vi "TEST-Get DataType Description String2.vi"() -> ()   [LabVIEW 2017]
panel:
  out "x = y?":bool[](array[boolean])
  out "unsigned byte array 2":u8[](array[numeric])
  out "unsigned byte array":u8[](array[numeric])
  out "variant 2":variant
  out "variant":variant
  out "Type 7":string
  out "Type 6":string
  out "Type 5":string
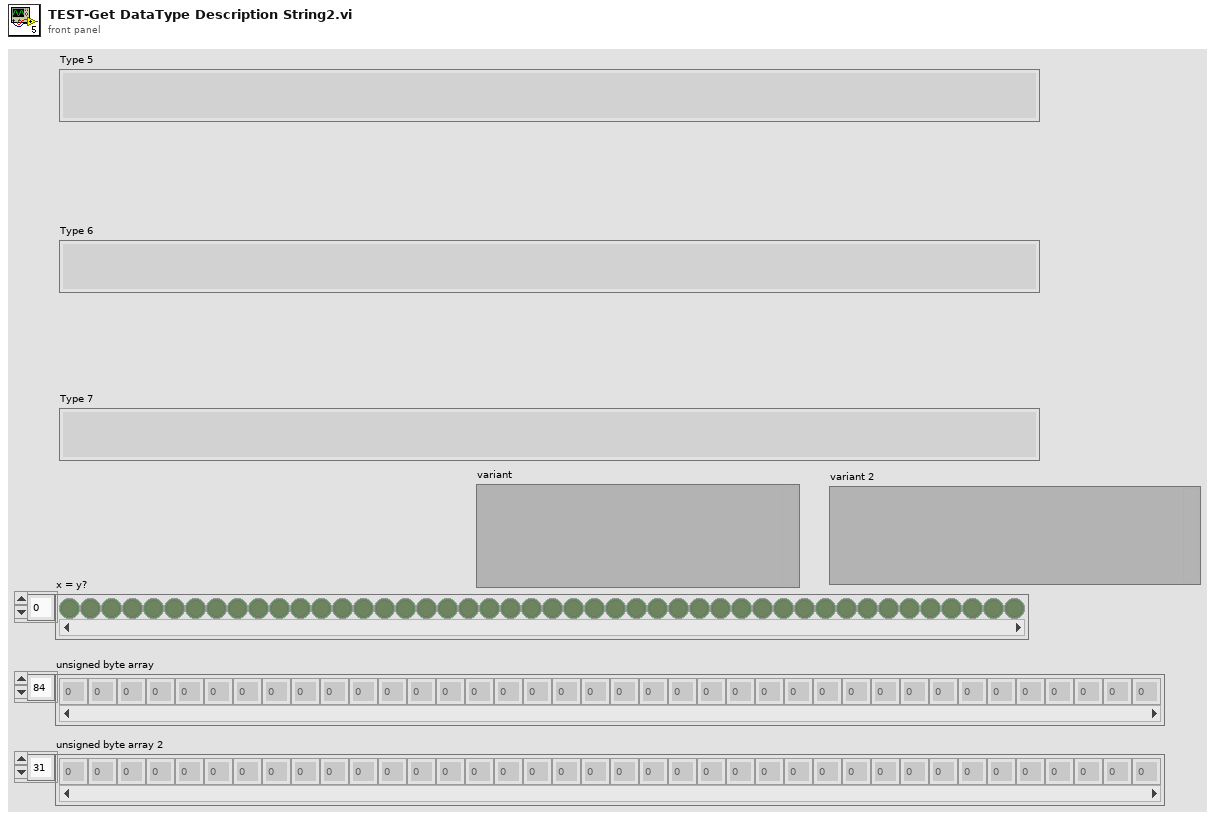
[diagram p1: front panel]
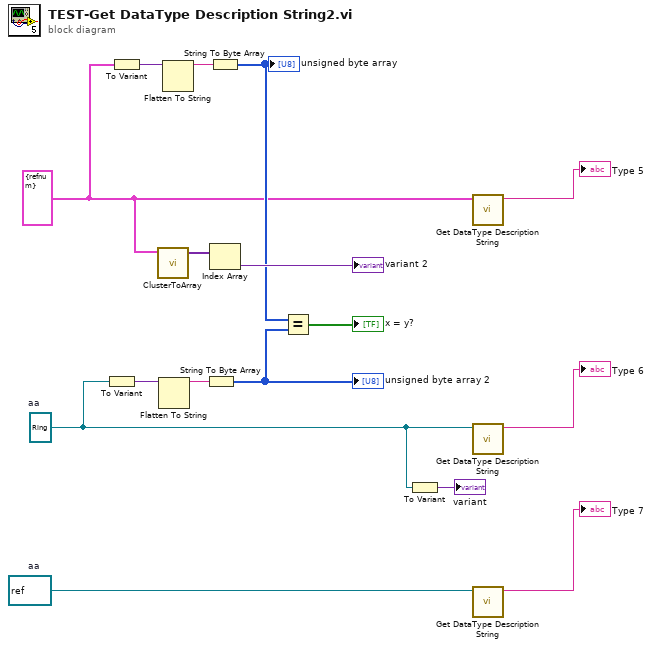
[diagram p0: block diagram]
diagram:
  w14 = refnum<k1> refnum items=["a", "b"]  # aa
  w5 = refnum<k1> refnum  # aa
  w1 = cluster{"aa":refnum<k1>} {"aa"=refnum} ("error in (no error)")
  n1 = To Variant(anything=w5) -> (Variant=w7:variant)
  n2 = To Variant(anything=w1) -> (Variant=w6:variant)
  n3 = call "ClusterToArray.vi"("Cluster"=w1) -> ("Array"=w12:variant[])  [unwired: 9 in, 1 out]
  n4 = Flatten To String(anything=w7) -> (data string=w8:string)  [unwired: 3 in, 2 out]
  n5 = Flatten To String(anything=w6) -> (data string=w9:string)  [unwired: 3 in, 2 out]
  n6 = String To Byte Array(string=w8) -> (unsigned byte array=w4:u8[])
  "unsigned byte array 2" <- w4
  n7 = String To Byte Array(string=w9) -> (unsigned byte array=w3:u8[])
  "unsigned byte array" <- w3
  n8 = Index Array(array=w12) -> (element=→"variant 2":variant)  [unwired: 1 in]
  n9 = Equal?(x=w3, y=w4) -> (x = y?=→"x = y?":bool[])
  n10 = To Variant(anything=w5) -> (Variant=→"variant":variant)
  n11 = call "Get DataType Description String.vi"("Variant"=w1) -> ("String"=→"Type 5":string)  [unwired: 9 in, 1 out]
  n12 = call "Get DataType Description String.vi"("Variant"=w5) -> ("String"=→"Type 6":string)  [unwired: 9 in, 1 out]
  n13 = call "Get DataType Description String.vi"("Variant"=w14) -> ("String"=→"Type 7":string)  [unwired: 9 in, 1 out]
